vi "CD Init_Prepare Async Data_MC Tx.vi"(8 "error in (no error)":errorcluster, 10 "Card Parameters (in)":T1, 11 "Channels In":T8[](array[typedef]) {"RTs"."Mode Codes"."Words Item Refs" format="%.0x"; "RTs"."Mode Codes"."Timestamp Channel Data Reference" format="%.0x"; "RTs"."subAddresses"."Words Item Refs" format="%.0x"; "RTs"."subAddresses"."Timestamp Channel Data Reference" format="%.0x"; "RTs"."Status Channel Data Reference" format="%.0x"; "RTs"."Command Channels Refs" format="%.0x"; "BC"."Acyclic Frames Trigger Channels Refs" format="%.0x"; "BC"."Command Channels Refs" format="%.0x"; "BC"."messages"."Timestamp Channel Data Reference" format="%.0x"; "BC"."messages"."Status Channel Data Refs" format="%.0x"; "BC"."messages"."Words Item Refs" format="%.0x"; "BC"."messages"."Words Block Data Refs"."Data Reference" format="%.0x"}) -> (0 "error out":errorcluster, 2 "Raw Values (RT to BC)":T3, 3 "Map (MC Tx)":T5[](array[typedef]) {"Word Data Reference" format="%.0x"})   [LabVIEW 2017, in "Ballard MIL-1553 Engine.lvlib"]
doc: "This VI creates a static association between NI-VS FIFO Channel Index and Physical Channel, Label Index, Parameter Index for Parameter Channel of a Tx Scheduled Label."
uses:
  Ballard MIL-1553 Engine.lvlib
  Shared/Controls and Global/RT Channel.ctl
  Shared/Controls and Global/RT BC.ctl
  <vilib>/NI Veristand/Custom Device API/Custom Device Item Ref.ctl
  Shared/Controls and Global/RT Message.ctl
  Shared/Controls and Global/RT messageType.ctl
  Shared/Controls and Global/RT CWD1.ctl
  Shared/Controls and Global/RT CWD2.ctl
  <vilib>/NI Veristand/Custom Device API/Data Reference.ctl
  <vilib>/NI Veristand/Custom Device API/Block Data Reference.ctl
  Shared/Controls and Global/RT Remote Terminal.ctl
  Shared/Controls and Global/RT Remote Terminal_rtMode.ctl
  Shared/Controls and Global/RT Remote Terminal_RT subAddress.ctl
  Shared/Controls and Global/RT Remote Terminal_RT direction.ctl
  Shared/Controls and Global/RT Remote Terminal_RT Mode Code.ctl
  Controls/RT Async_Map RT2BC.ctl
  Controls/RT Async_Map_Type.ctl
  Controls/RT Async_Raw Values.ctl
  Controls/RT Async_Raw Values to Messages Index_Association.ctl
  Controls/Card Parameters.ctl
  Shared/Controls and Global/Initialization Method.ctl
  Controls/RT Async_Raw Values_Association.ctl
  <instrlib>/BTI1553Lib/Public/Controls/1553 RT Transfer Type.ctl
  <instrlib>/BTI1553Lib/Public/Controls/1553 Transfer Direction.ctl
  <instrlib>/BTI1553Lib/Private/RT/Configure/Get RT Xfer Handle.vi
  <vilib>/NI VeriStand/Custom Device API/Custom Device API.lvlib
  <instrlib>/BTI1553Lib/BTI1553LV.lvlib
  Shared/Ballard 1553 Shared.lvlib
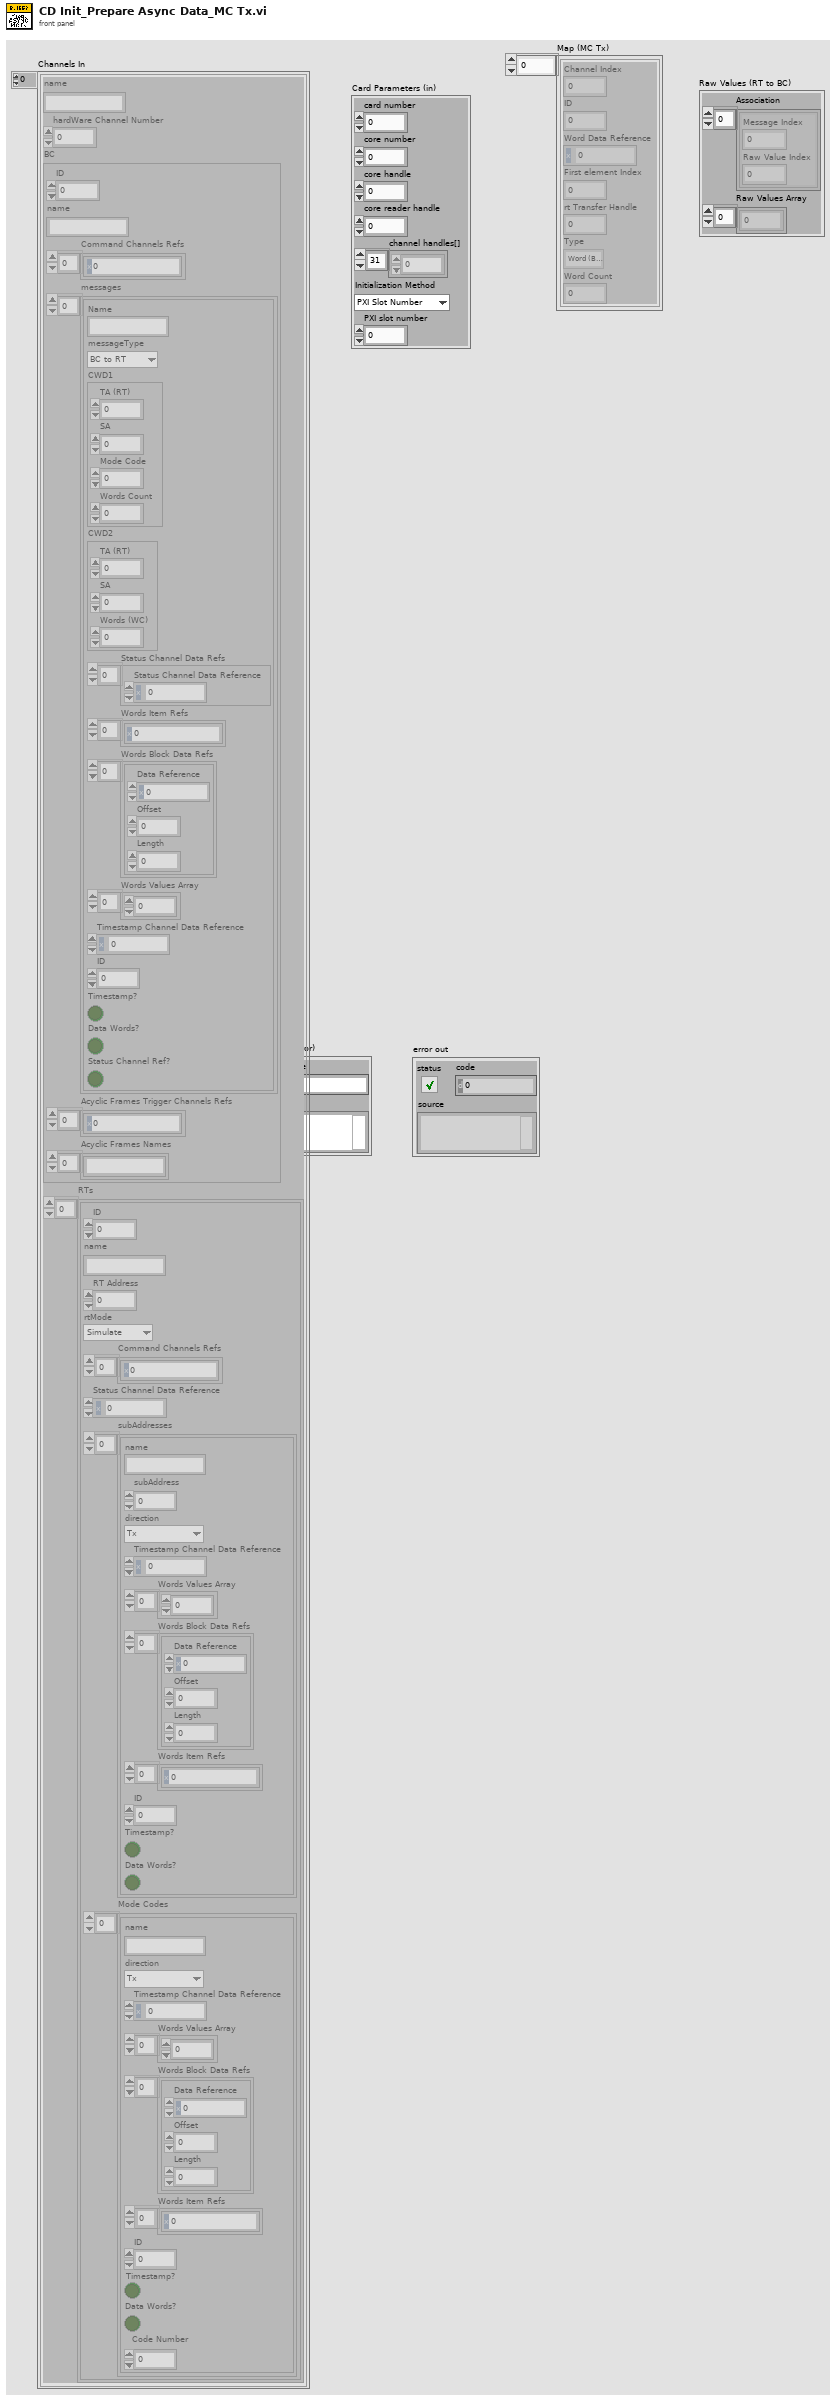
[diagram p1: front panel]
types:
  T1 = typedef "Ballard MIL-1553 Engine.lvlib/Card Parameters.ctl" = cluster{"card number":i32, "core number":i32, "core handle":u64, "core reader handle":u64, "channel handles[]":u64[], "Initialization Method":T2, "PXI slot number":i32}
  T2 = typedef "Ballard 1553 Shared.lvlib/Initialization Method.ctl" = enum16{"PXI Slot Number", "Card Number"}
  T3 = typedef "Ballard MIL-1553 Engine.lvlib/RT Async_Raw Values.ctl" = cluster{"Association":T4[], "Raw Values Array":u16[]}
  T4 = typedef "Ballard MIL-1553 Engine.lvlib/RT Async_Raw Values to Messages Index_Association.ctl" = cluster{"Message Index":i32, "Raw Value Index":i32}
  T5 = typedef "Ballard MIL-1553 Engine.lvlib/RT Async_Map RT2BC.ctl" = cluster{"Channel Index":i32, "ID":i32, "Word Data Reference":T6, "First element Index":i32, "rt Transfer Handle":u64, "Type":T7, "Word Count":i32}
  T6 = typedef "Custom Device API.lvlib/Data Reference.ctl" = i32
  T7 = typedef "Ballard MIL-1553 Engine.lvlib/RT Async_Map_Type.ctl" = enum16{"Word (BC to RT)", "Word (MC (Rx))", "Acyclic Message Trigger", "Word (RT to ..)", "Word (RT to RT)", "Word (MC (Tx))", "RT Status", "BC Commands", "RT Commands"}
  T8 = typedef "Ballard 1553 Shared.lvlib/RT Channel.ctl" = cluster{"name":string, "hardWare Channel Number":u16, "BC":T9, "RTs":T16[]}
  T9 = typedef "Ballard 1553 Shared.lvlib/RT BC.ctl" = cluster{"ID":i32, "name":string, "Command Channels Refs":T10[], "messages":T11[], "Acyclic Frames Trigger Channels Refs":T10[], "Acyclic Frames Names":string[]}
  T10 = typedef "Custom Device API.lvlib/Custom Device Item Ref.ctl" = u64
  T11 = typedef "Ballard 1553 Shared.lvlib/RT Message.ctl" = cluster{"Name":string, "messageType":T12, "CWD1":T13, "CWD2":T14, "Status Channel Data Refs":T6[], "Words Item Refs":T10[], "Words Block Data Refs":T15[], "Words Values Array":u16[], "Timestamp Channel Data Reference":T6, "ID":i32, "Timestamp?":bool, "Data Words?":bool, "Status Channel Ref?":bool}
  T12 = typedef "Ballard 1553 Shared.lvlib/RT messageType.ctl" = enum16{"BC to RT", "RT to BC", "RT to RT", "MC (Rx)", "MC (Tx)"}
  T13 = typedef "Ballard 1553 Shared.lvlib/RT CWD1.ctl" = cluster{"TA (RT)":i8, "SA":i8, "Mode Code":i8, "Words Count":i8}
  T14 = typedef "Ballard 1553 Shared.lvlib/RT CWD2.ctl" = cluster{"TA (RT)":i8, "SA":i8, "Words (WC)":i8}
  T15 = typedef "Custom Device API.lvlib/Block Data Reference.ctl" = cluster{"Data Reference":T6, "Offset":u64, "Length":u64}
  T16 = typedef "Ballard 1553 Shared.lvlib/RT Remote Terminal.ctl" = cluster{"ID":i32, "name":string, "RT Address":i32, "rtMode":T17, "Command Channels Refs":T10[], "Status Channel Data Reference":T6, "subAddresses":T18[], "Mode Codes":T20[]}
  T17 = typedef "Ballard 1553 Shared.lvlib/RT Remote Terminal_rtMode.ctl" = enum16{"Simulate", "Monitor", "Disable"}
  T18 = typedef "Ballard 1553 Shared.lvlib/RT Remote Terminal_RT subAddress.ctl" = cluster{"name":string, "subAddress":i8, "direction":T19, "Timestamp Channel Data Reference":T6, "Words Values Array":u16[], "Words Block Data Refs":T15[], "Words Item Refs":T10[], "ID":i32, "Timestamp?":bool, "Data Words?":bool}
  T19 = typedef "Ballard 1553 Shared.lvlib/RT Remote Terminal_RT direction.ctl" = enum16{"Tx", "Rx"}
  T20 = typedef "Ballard 1553 Shared.lvlib/RT Remote Terminal_RT Mode Code.ctl" = cluster{"name":string, "direction":T19, "Timestamp Channel Data Reference":T6, "Words Values Array":u16[], "Words Block Data Refs":T15[], "Words Item Refs":T10[], "ID":i32, "Timestamp?":bool, "Data Words?":bool, "Code Number":i32}
  T21 = typedef "Ballard MIL-1553 Engine.lvlib/RT Async_Raw Values_Association.ctl" = cluster{"Channel Data Reference":T6, "Raw Value Index":i32}
  T22 = typedef "BTI1553LV.lvlib/1553 Transfer Direction.ctl" = u32
  T23 = typedef "BTI1553LV.lvlib/1553 RT Transfer Type.ctl" = u32
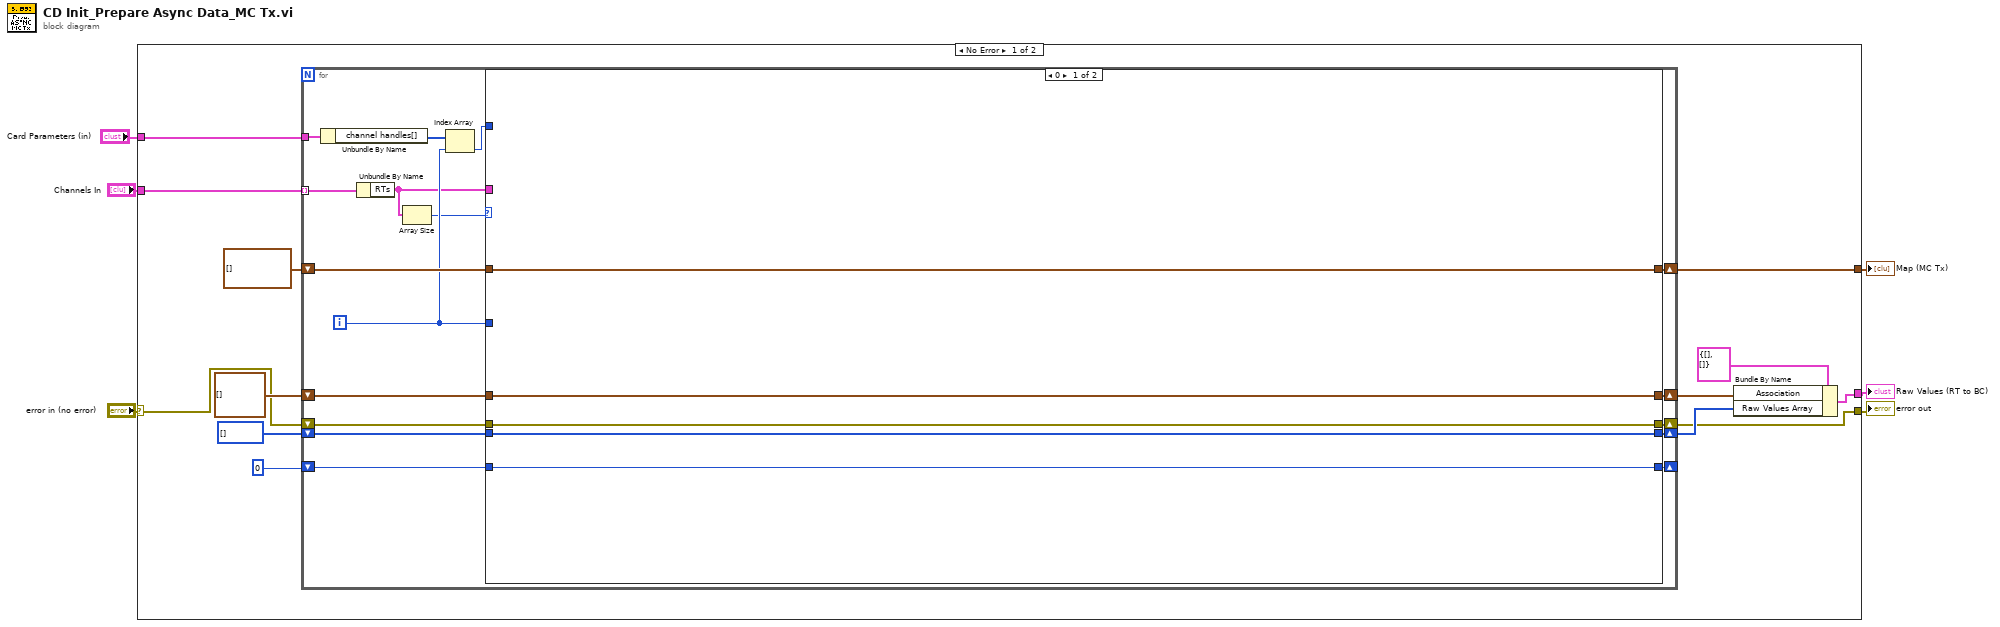
[diagram p0: block diagram]
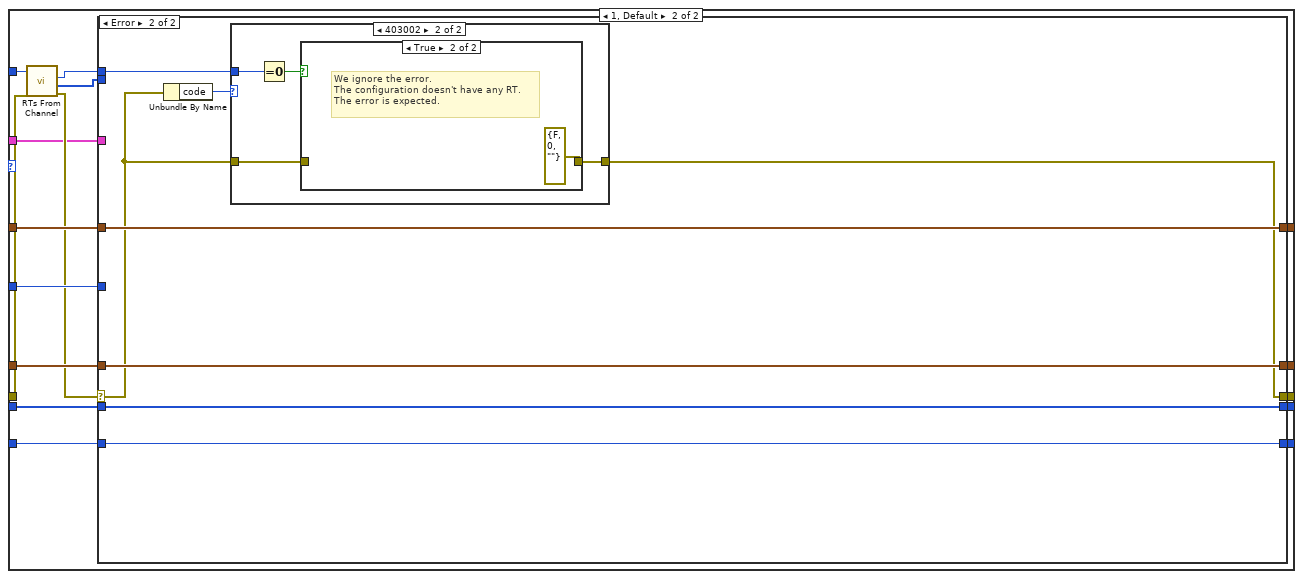
[diagram p2: hidden frame]
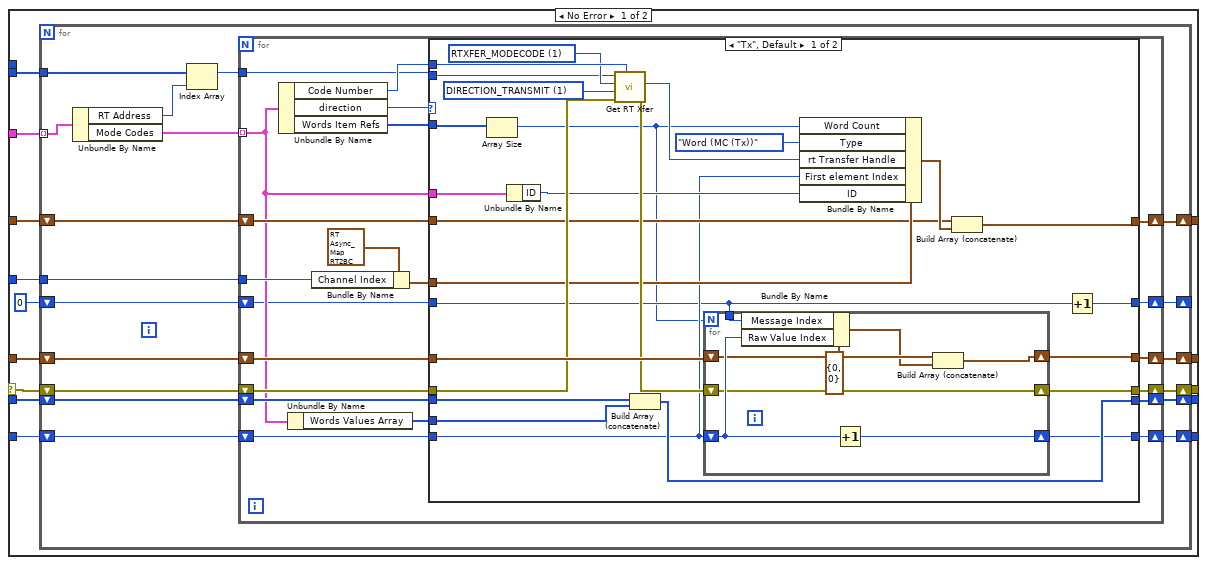
[diagram p3: hidden frame]
diagram:
  n1 = case shown="No Error" "error in (no error)" {
    selector: "error in (no error)" -> [w8 w166]
    tunnel: [w7 w166] -> w5
    tunnel: "Channels In" -> [w19 _]
    tunnel: [w17 _] -> w3
    tunnel: [w13 _] -> w2
    tunnel: "Card Parameters (in)" -> [w9 _]
    frame No Error {
      n2 = for {
        tunnel: w19 -> [w36] mode=indexing
        shift-right: [w34] -> w17
        shift-left: T5[] [] -> [w35]
        shift-right: [w32] -> w14
        shift-left: T21[] [] -> [w33]
        shift-right: [w28] -> w11
        shift-left: u16[] [] -> [w31]
        shift-right: [w29] -> _
        shift-left: 0 -> [w30]
        tunnel: w9 -> [w27]
        shift-right: [w24] -> w7
        shift-left: w8 -> [w22]
        i -> [w25]
        n3 = Unbundle By Name(w27) -> ("channel handles[]"=w26:u64[])
        n4 = Unbundle By Name(w36) -> ("RTs"=w21:T16[])
        n5 = Array Size(array=w21) -> (size(s)=w20:i32)
        n6 = Index Array(array=w26, index=w25) -> (element=w23:u64)
        n7 = case shown="0" w20 {
          tunnel: w35 -> [w41 w57]
          tunnel: [w41 w56] -> w34
          tunnel: w33 -> [w40 w55]
          tunnel: [w40 w54] -> w32
          tunnel: w31 -> [w38 w53]
          tunnel: w30 -> [w37 w52]
          tunnel: [w37 w51] -> w29
          tunnel: [w38 w50] -> w28
          tunnel: w25 -> [_ w49]
          tunnel: [w39 w48] -> w24
          tunnel: w23 -> [_ w47]
          tunnel: w22 -> [w39 w46]
          tunnel: w21 -> [_ w42]
          frame 0 {
          }
          frame 1, Default {
            n8 = call <instrlib>:"RTs From Channel.vi"("error in (no error)"=w46, "channel handle in"=w47) -> ("error out"=w44:errorcluster, "remote terminal handles out"=w45:u64[], "remote terminal count out"=w43:i32)  [unwired: 6 in, 1 out]
            n9 = case shown="Error" w44 {
              selector: w44 -> [w58 w153]
              tunnel: w42 -> [w71 _]
              tunnel: w57 -> [w70 w155]
              tunnel: [w69 w155] -> w56
              tunnel: w55 -> [w68 w156]
              tunnel: [w67 w156] -> w54
              tunnel: w53 -> [w66 w157]
              tunnel: w52 -> [w65 w158]
              tunnel: [w64 w158] -> w51
              tunnel: [w63 w157] -> w50
              tunnel: w49 -> [w62 _]
              tunnel: [w61 w151] -> w48
              tunnel: w45 -> [w60 _]
              tunnel: w43 -> [_ w152]
              frame No Error {
                n10 = for {
                  tunnel: w71 -> [w76] mode=indexing
                  shift-right: [w87] -> w69
                  shift-left: w70 -> [w88]
                  tunnel: w62 -> [w89]
                  shift-right: [w86] -> w67
                  shift-left: w68 -> [w82]
                  shift-right: [w85] -> w63
                  shift-left: w66 -> [w81]
                  shift-right: [w84] -> w64
                  shift-left: w65 -> [w83]
                  tunnel: w60 -> [w80]
                  shift-right: [w78] -> w61
                  shift-left: w58 -> [w79]
                  shift-right: [w72] -> _
                  shift-left: 0 -> [w73]
                  n11 = Unbundle By Name(w76) -> ("RT Address"=w74:i32, "Mode Codes"=w77:T20[])
                  n12 = Index Array(array=w80, index=w74) -> (element=w75:u64)
                  n13 = for {
                    tunnel: w89 -> [w110]
                    tunnel: w77 -> [w93] mode=indexing
                    tunnel: w75 -> [w95]
                    shift-right: [w103] -> w84
                    shift-left: w83 -> [w102]
                    shift-right: [w97] -> w78
                    shift-left: w79 -> [w98]
                    shift-right: [w108] -> w87
                    shift-left: w88 -> [w109]
                    shift-right: [w105] -> w86
                    shift-left: w82 -> [w101]
                    shift-right: [w104] -> w85
                    shift-left: w81 -> [w100]
                    shift-right: [w90] -> w72
                    shift-left: w73 -> [w91]
                    n14 = Unbundle By Name(w93) -> ("Code Number"=w96:i32, "direction"=w92:T19, "Words Item Refs"=w106:T10[])
                    n15 = Unbundle By Name(w93) -> ("Words Values Array"=w99:u16[])
                    n16 = Bundle By Name(cluster=T5 {"Channel Index"=0, "ID"=0, "Word Data Reference"=0, "First element Index"=0, "rt Transfer Handle"=0, "Type"=enum."Word (BC to RT)", "Word Count"=0} ("Association"), "Channel Index"=w110) -> (w107:T5)
                    n17 = case shown="\"Tx\", Default" w92 {
                      tunnel: w109 -> [w117 w150]
                      tunnel: [w116 w150] -> w108
                      tunnel: w107 -> [w122 _]
                      tunnel: w106 -> [w114 _]
                      tunnel: [w123 w149] -> w105
                      tunnel: [w136 w147] -> w104
                      tunnel: [w135 w146] -> w103
                      tunnel: w102 -> [w113 w146]
                      tunnel: w101 -> [w134 w149]
                      tunnel: w100 -> [w133 w147]
                      tunnel: w99 -> [w132 _]
                      tunnel: w98 -> [w131 w148]
                      tunnel: [w129 w148] -> w97
                      tunnel: w96 -> [w128 _]
                      tunnel: w95 -> [w126 _]
                      tunnel: w93 -> [w125 _]
                      tunnel: w91 -> [w112 w145]
                      tunnel: [w115 w145] -> w90
                      frame "Tx", Default {
                        w124 = T22 1 items=["DIRECTION_RECEIVE", "DIRECTION_TRANSMIT"] ("transfer direction")
                        w127 = T23 1 items=["RTXFER_SUBADDRESS", "RTXFER_MODECODE"] ("transfer type")
                        n18 = Array Size(array=w114) -> (size(s)=w111:i32)
                        n19 = Unbundle By Name(w125) -> ("ID"=w119:i32)
                        n20 = call-poly <instrlib>:"Get RT Xfer.vi"("transfer sa number or mc number"=w128, "error in (no error)"=w131, "transfer direction"=w124, "transfer type"=w127, "remote terminal handle in"=w126) -> ("error out"=w130:errorcluster, "rt transfer handle out"=w120:u64)  [unwired: 4 in, 1 out]
                        n21 = Build Array (concatenate)(w133, w132) -> (w136:u16[])
                        n22 = for {
                          N: w111 -> [_]
                          shift-right: [w144] -> w135
                          shift-left: w113 -> [w143]
                          shift-right: [w141] -> w129
                          shift-left: w130 -> [w141]
                          shift-right: [w138] -> w123
                          shift-left: w134 -> [w142]
                          tunnel: w112 -> [w137]
                          n23 = Bundle By Name(cluster=T4 {"Message Index"=0, "Raw Value Index"=0}, "Message Index"=w137, "Raw Value Index"=w143) -> (w139:T4)
                          n24 = Increment(x=w143) -> (x+1=w144:i32)
                          n25 = Build Array (concatenate)(w142, w139) -> (w138:T21[])
                        }
                        n26 = Bundle By Name(cluster=w122, "Word Count"=w111, "Type"=RT_Async_Map_Type."Word (MC (Tx))", "rt Transfer Handle"=w120, "First element Index"=w113, "ID"=w119) -> (w118:T5)
                        n27 = Build Array (concatenate)(w117, w118) -> (w116:T5[])
                        n28 = Increment(x=w112) -> (x+1=w115:i32)
                      }
                      frame "Rx" {
                      }
                    }
                  }
                }
              }
              frame Error {
                n29 = Unbundle By Name(w153) -> ("code"=w154:i32)
                n30 = case shown="403002" w154 {
                  tunnel: w153 -> [w159 w161]
                  tunnel: w152 -> [_ w163]
                  tunnel: [w159 w160] -> w151
                  frame 0, Default {
                  }
                  frame 403002 {
                    n31 = Equal To 0?(x=w163) -> (x = 0?=w162:bool)
                    n32 = case shown="True" w162 {
                      tunnel: w161 -> [w164 _]
                      tunnel: [w164 errorcluster {"status"=FALSE, "code"=0, "source"=""} ("error IO")] -> w160
                      frame False {
                      }
                      frame True {
                        # "We ignore the error.\nThe configuration doesn't have any RT.\nThe error is expected."
                      }
                    }
                  }
                }
              }
            }
          }
        }
      }
      n33 = Bundle By Name(cluster=T3 {"Association"=[], "Raw Values Array"=[]} ("Raw Values"), "Association"=w14, "Raw Values Array"=w11) -> (w13:T3)
    }
    frame Error {
    }
  }
  "error out" <- w5
  "Map (MC Tx)" <- w3
  "Raw Values (RT to BC)" <- w2
